vi "Unload Project.vi"(8 "error in (no error)":errorcluster, 11 "Project Loader In":refnum<class "Project Loader.lvclass">) -> (0 "error out":errorcluster, 3 "Project Loader Out":refnum<class "Project Loader.lvclass">)   [LabVIEW 2020, in "Project Loader.lvclass"]
uses:
  Project Loader.lvclass
  Project Loader.lvclass/Project Loader.ctl
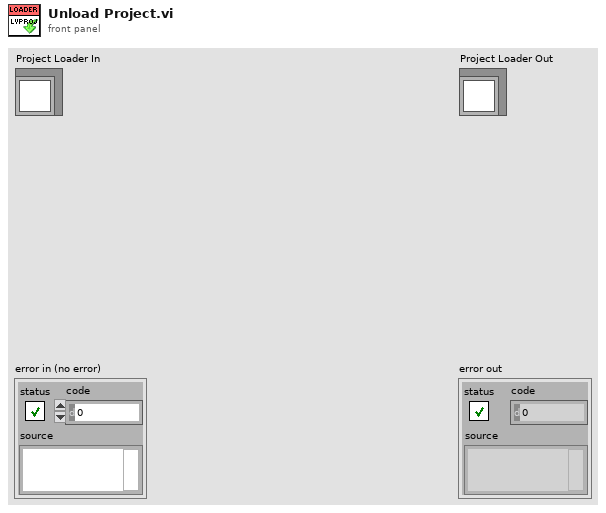
[diagram p1: front panel]
types:
  T1 = enum32{"Invalid", "Standard", "Closed", "Hidden", "Minimized", "Maximized"}
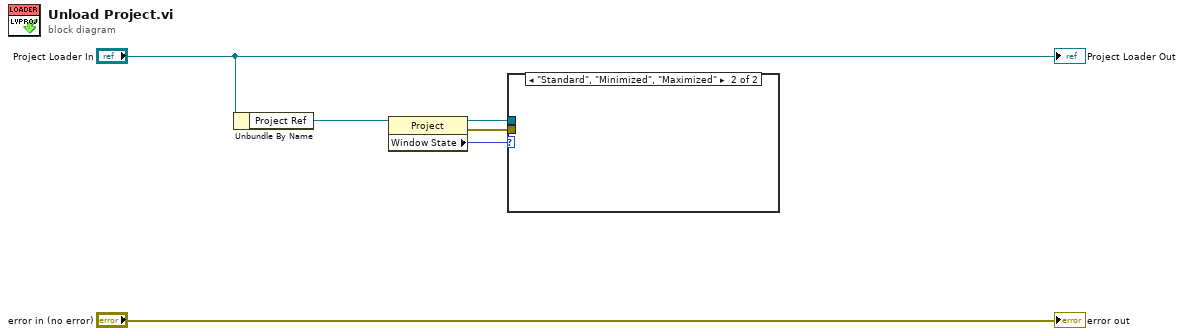
[diagram p0: block diagram]
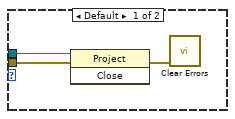
[diagram p2: hidden frame]
diagram:
  n1 = Unbundle By Name("Project Loader In") -> ("Project Ref"=w4:refnum<vi>)
  n2 = property class="Project"(reference=w4) -> (reference out=w3:refnum<vi>, error out=w1:errorcluster, "Window State"=w2:T1)  [unwired: 1 in]
  n3 = case shown="\"Standard\", \"Minimized\", \"Maximized\"" w2 {
    tunnel: w3 -> [w8 _]
    tunnel: w1 -> [w7 _]
    frame Default {
      n4 = invoke class="Project" method="Close"(reference=w8, error in=w7) -> (error out=w9:errorcluster)  [unwired: 1 in, 2 out]
      n5 = call <vilib>:"Clear Errors.vi"("error in (no error)"=w9) -> ()  [unwired: 5 in, 2 out]
    }
    frame "Standard", "Minimized", "Maximized" {
    }
  }
  "error out" <- "error in (no error)"
  "Project Loader Out" <- "Project Loader In"
